vi "Main.vi"(8 "error in":errorcluster, 11 "Message Pump":refnum<class "Message Pump.lvclass">) -> (0 "error out":errorcluster, 3 "Message Pump out":refnum<class "Message Pump.lvclass">)   [LabVIEW 2023, in "Message Pump.lvclass"]
uses:
  Message Pump.lvclass
  C:/Program Files (x86)/National Instruments/LabVIEW 2023/vi.lib/addons/_Workers/Library/Classes/Worker/Worker.lvclass
  <vilib>/addons/_Workers/Library/Classes/Message Queue/Message Queue.lvclass
  <vilib>/addons/_Workers/Library/Case Label.ctl
  Message Pump.lvclass/Message Pump.ctl
  Initialization Data.ctl
  <vilib>/Utility/error.llb/Error Cluster From Error Code.vi
  <vilib>/addons/_Workers/Library/Classes/Message/Enqueue Message to Queue - Silent Mode.vi
  <vilib>/ErrorRing/Error Ring.xnode
  <vilib>/addons/_Workers/Library/Classes/Worker/Worker.lvclass
  <vilib>/addons/_Workers/Library/Workers.lvlib
  <vilib>/addons/_Workers/Library/Classes/Message/Message.lvclass
  C:/Program Files (x86)/National Instruments/LabVIEW 2023/vi.lib/addons/_Workers/Library/Classes/Workers Object/Workers Object.lvclass
  C:/Projects/DPP Workers/Workers/Message Pump/Message Pump.lvclass
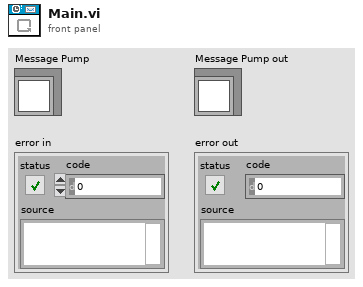
[diagram p1: front panel]
types:
  T1 = typedef "Message Pump.lvclass/Initialization Data.ctl" = cluster{"Caller Queue":refnum<class "Message Queue.lvclass">}
  T2 = typedef "WORKERS.lvlib/Case Label.ctl" = string
  T3 = typedef "Workers.lvlib/Case Label.ctl" = string
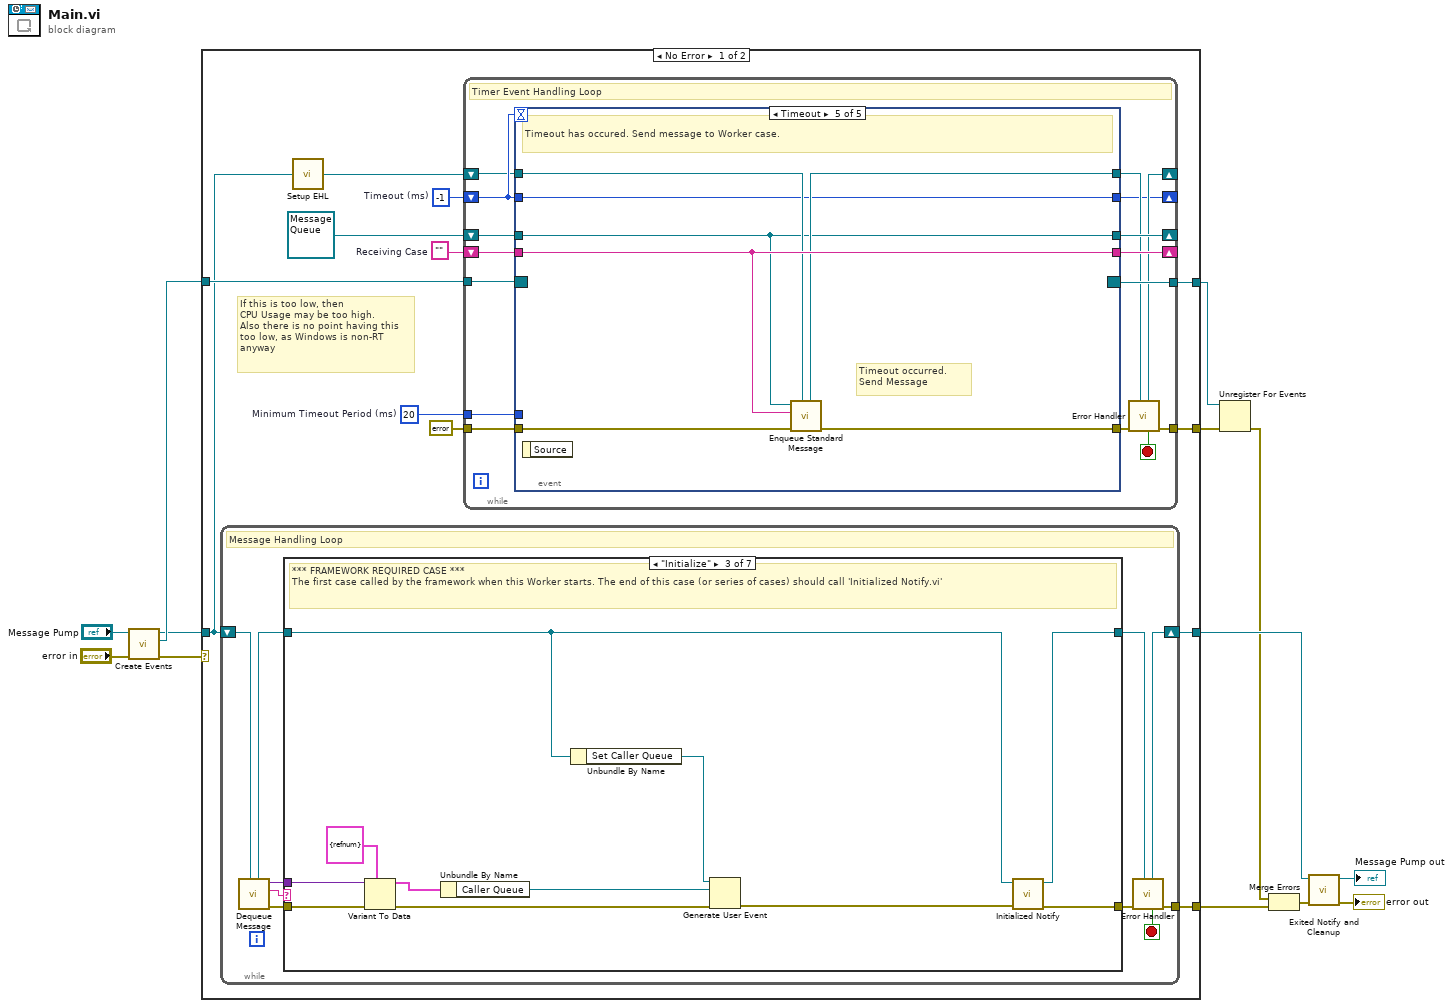
[diagram p0: block diagram]
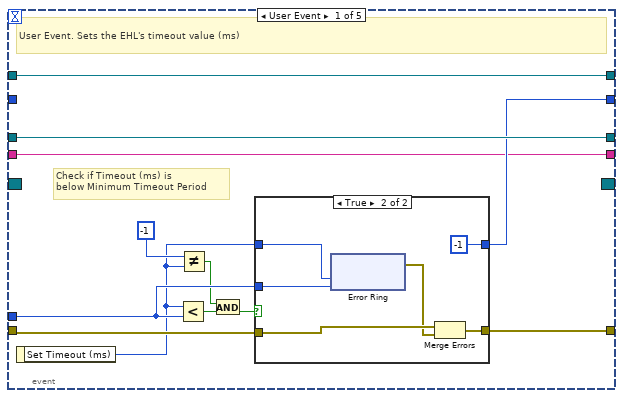
[diagram p2: hidden frame]
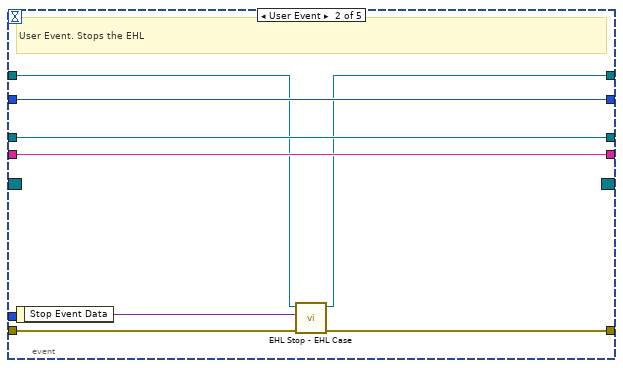
[diagram p4: hidden frame]
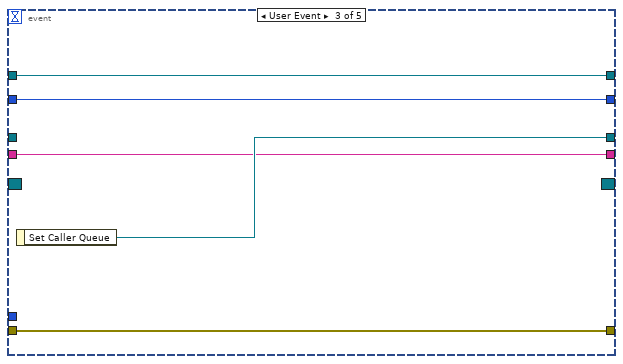
[diagram p5: hidden frame]
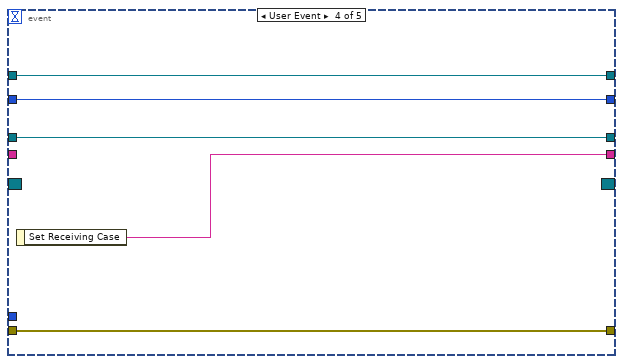
[diagram p6: hidden frame]
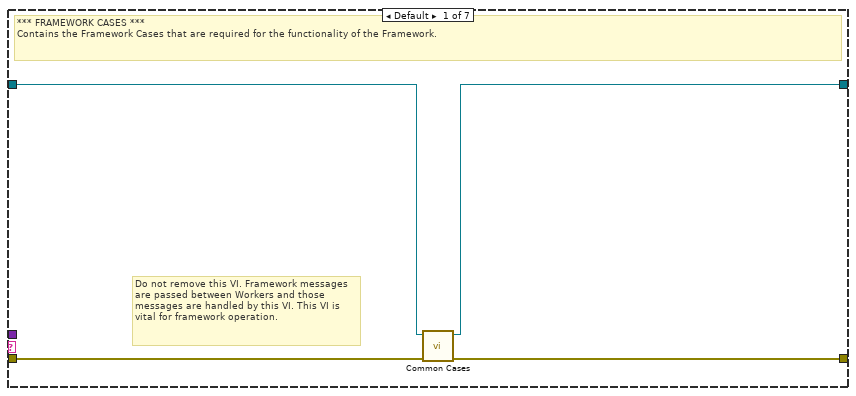
[diagram p7: hidden frame]
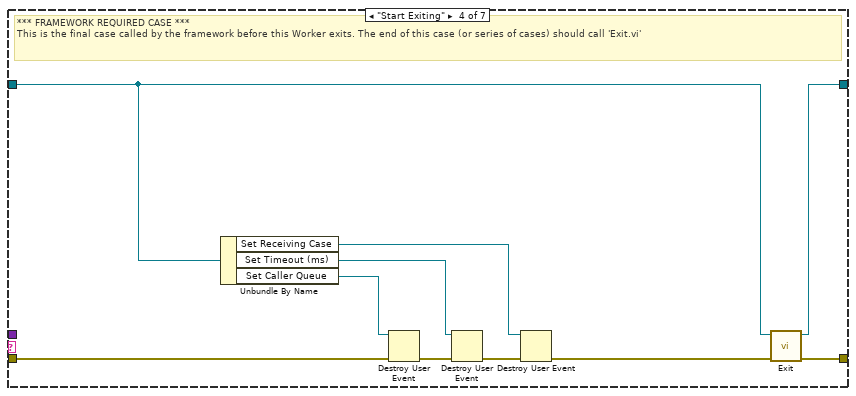
[diagram p9: hidden frame]
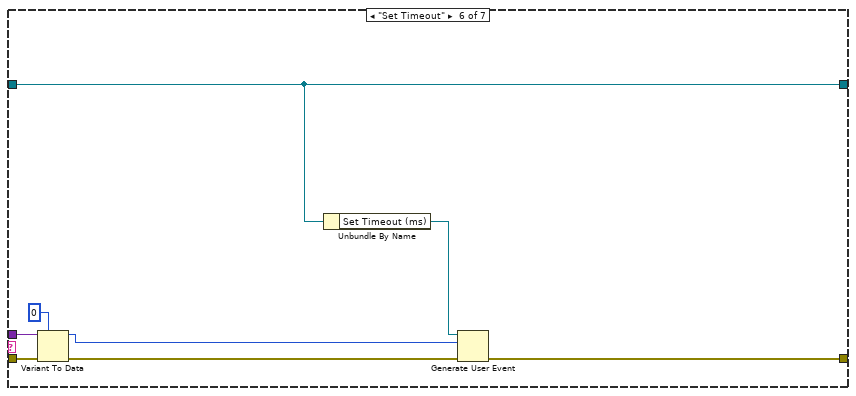
[diagram p11: hidden frame]
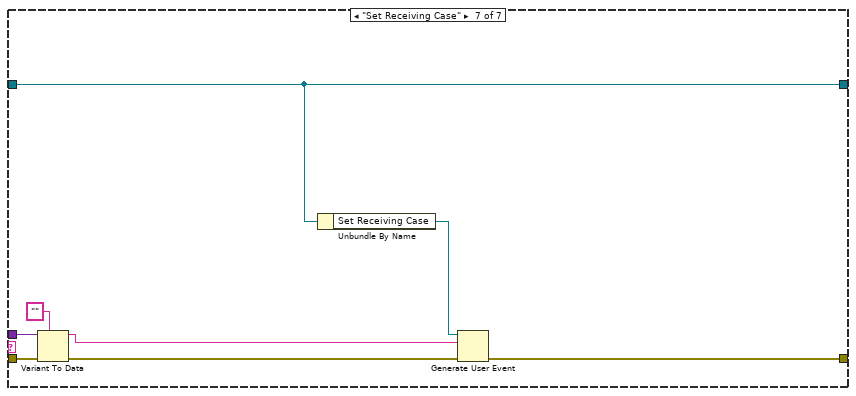
[diagram p12: hidden frame]
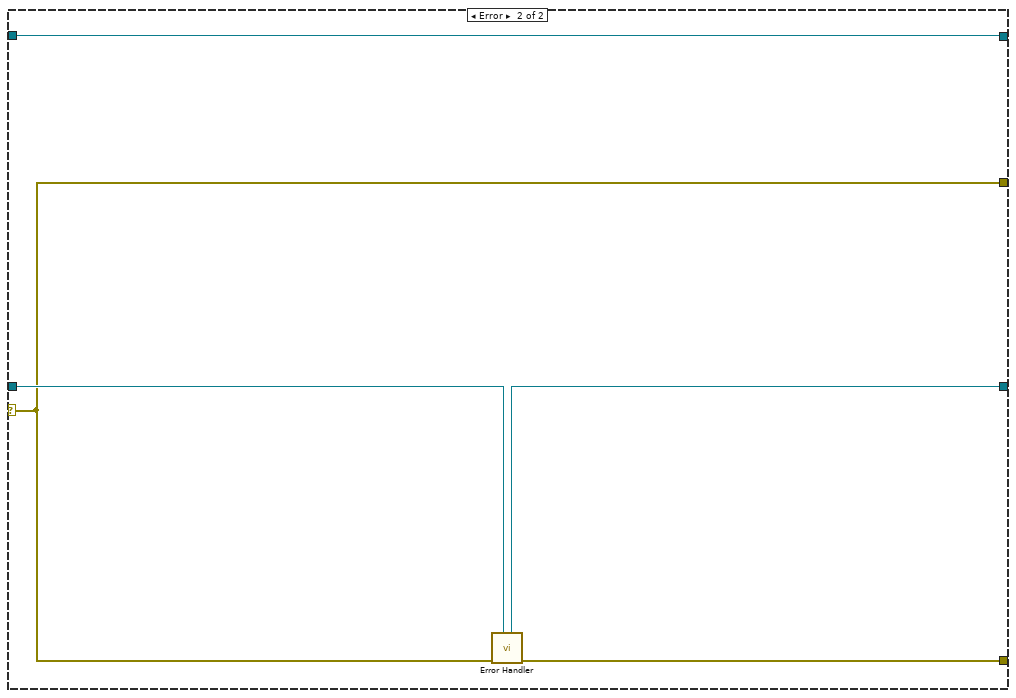
[diagram p13: hidden frame]
diagram:
  n1 = call "Create Events.vi"("error in"="error in", "Message Pump in"="Message Pump") -> ("error out"=w8:errorcluster, "Event Registration Refnum"=w9:refnum<event-registration>, "Message Pump out"=w4:refnum<class "Message Pump.lvclass">)  [unwired: 6 in]
  n2 = case shown="No Error" w8 {
    tunnel: w4 -> [w15 w153]
    tunnel: [w25 w154] -> w12
    tunnel: [w24 w152] -> w13
    selector: w8 -> [_ w151]
    tunnel: [w17 w151] -> w2
    tunnel: [w19 w150] -> w3
    tunnel: w9 -> [w18 w150]
    frame No Error {
      w23 = T2 ""  # Receiving Case
      w22 = 20  # Minimum Timeout Period (ms)
      w21 = -1  # Timeout (ms)
      # "If this is too low, then \nCPU Usage may be too high.\nAlso there is no point having this\ntoo low, as Windows is non-RT\nanyway"
      n3 = while {
        shift-right: [w102] -> w24
        shift-left: w15 -> [w104]
        tunnel: [w103] -> w25
        stop <- w95 stop-if-true
        # "Message Handling Loop"
        n4 = call-dynamic "Dequeue Message.vi"("Worker"=w104) -> ("error out"=w101:errorcluster, "Case out"=w96:string, "Data out"=w97:variant, "Worker out"=w99:refnum<class "Message Pump.lvclass">)  [unwired: 6 in, 1 out]
        n5 = case "WORKERS MHL Case Structure (DO NOT CHANGE LABEL NAME)" shown="\"Initialize\"" w96 {
          tunnel: w101 -> [w108 w109 w119 w124 w132 w141 w149]
          tunnel: [w107 w109 w121 w131 w132 w137 w146] -> w100
          tunnel: w99 -> [w106 w110 w113 w122 w133 w135 w144]
          tunnel: [w105 w110 w120 w130 w133 w135 w144] -> w98
          tunnel: w97 -> [_ _ w118 _ _ w140 w148]
          frame Default {
            # "Do not remove this VI. Framework messages are passed between Workers and those messages are handled by this VI. This VI is vital for framework operation."
            # "*** FRAMEWORK CASES ***\nContains the Framework Cases that are required for the functionality of the Framework."
            n6 = call-dynamic "Common Cases.vi"("error in"=w108, "Worker in"=w106) -> ("error out"=w107:errorcluster, "Worker out"=w105:refnum<class "Message Pump.lvclass">)  [unwired: 8 in]
          }
          frame "------ FRAMEWORK REQUIRED CASES ------" {
            # "Start of Framework Required Cases"
          }
          frame "Initialize" {
            # "*** FRAMEWORK REQUIRED CASE ***\nThe first case called by the framework when this Worker starts. The end of this case (or series of cases) should call 'Initialized Notify.vi'"
            n7 = Variant To Data(error in=w119, type=T1 {"Caller Queue"=refnum} ("Initialize Data"), Variant=w118) -> (data=w116:T1, error out=w115:errorcluster)
            n8 = Unbundle By Name(w116) -> ("Caller Queue"=w111:refnum<class "Message Queue.lvclass">)
            n9 = Unbundle By Name(w113) -> ("Set Caller Queue"=w114:refnum<user-event>)
            n10 = Generate User Event(user event=w114, event data cluster=w111, error in=w115) -> (error out=w112:errorcluster)  [unwired: 1 in, 1 out]
            n11 = call-dynamic "Initialized Notify.vi"("error in"=w112, "Worker"=w113) -> ("error out"=w121:errorcluster, "dup Worker out"=w120:refnum<class "Message Pump.lvclass">)  [unwired: 8 in]
          }
          frame "Start Exiting" {
            # "*** FRAMEWORK REQUIRED CASE ***\nThis is the final case called by the framework before this Worker exits. The end of this case (or series of cases) should call 'Exit.vi'"
            n12 = Unbundle By Name(w122) -> ("Set Receiving Case"=w129:refnum<user-event>, "Set Timeout (ms)"=w125:refnum<user-event>, "Set Caller Queue"=w126:refnum<user-event>)
            n13 = Destroy User Event(user event=w126, error in=w124) -> (error out=w127:errorcluster)
            n14 = Destroy User Event(user event=w125, error in=w127) -> (error out=w128:errorcluster)
            n15 = Destroy User Event(user event=w129, error in=w128) -> (error out=w123:errorcluster)
            n16 = call-dynamic "Exit.vi"("error_in"=w123, "Worker"=w122) -> ("error out"=w131:errorcluster, "dup Worker out"=w130:refnum<class "Message Pump.lvclass">)  [unwired: 8 in]
          }
          frame "-----------------------------------------------" {
            # "End of Framework Required Cases"
          }
          frame "Set Timeout" {
            n17 = Variant To Data(error in=w141, type=0 ("Timeout (ms)"), Variant=w140) -> (data=w134:i32, error out=w136:errorcluster)
            n18 = Unbundle By Name(w135) -> ("Set Timeout (ms)"=w138:refnum<user-event>)
            n19 = Generate User Event(user event=w138, event data cluster=w134, error in=w136) -> (error out=w137:errorcluster)  [unwired: 1 in, 1 out]
          }
          frame "Set Receiving Case" {
            n20 = Variant To Data(error in=w149, type=T2 "" ("Receiving Case"), Variant=w148) -> (data=w143:T2, error out=w145:errorcluster)
            n21 = Unbundle By Name(w144) -> ("Set Receiving Case"=w147:refnum<user-event>)
            n22 = Generate User Event(user event=w147, event data cluster=w143, error in=w145) -> (error out=w146:errorcluster)  [unwired: 1 in, 1 out]
          }
        }
        n23 = call-dynamic "Error Handler.vi"("Worker"=w98, "error_in"=w100) -> ("error out"=w103:errorcluster, "Stop Loop"=w95:bool, "Worker out"=w102:refnum<class "Message Pump.lvclass">)  [unwired: 7 in]
      }
      n24 = call-dynamic "Setup EHL.vi"("Worker"=w15) -> ("Worker out"=w14:refnum<class "Message Pump.lvclass">)  [unwired: 14 in]
      n25 = while "Event Handling Loop" {
        shift-right: [w26] -> _
        shift-left: w21 -> [w40]
        tunnel: errorcluster {"status"=FALSE, "code"=0, "source"=""} ("error IO") -> [w41]
        tunnel: [w31] -> w17
        shift-right: [w37] -> _
        shift-left: refnum<class "Message Queue.lvclass"> refnum ("Worker Queue") -> [w38]
        shift-right: [w36] -> _
        shift-left: w23 -> [w39]
        tunnel: w18 -> [w35]
        tunnel: [w34] -> w19
        tunnel: w22 -> [w33]
        shift-right: [w28] -> _
        shift-left: w14 -> [w30]
        stop <- w27 stop-if-true
        # "Timer Event Handling Loop"
        n26 = event shown="[4] Timeout" {
          selector: w35 -> [_ _ _ _ _]
          dyn-events: [_ _ _ _ _] -> w34
          timeout: w40 -> [_ _ _ _ _]
          tunnel: w41 -> [w50 w77 w82 w87 w94]
          tunnel: [w51 w73 w82 w87 w92] -> w32
          tunnel: w40 -> [_ w76 w81 w86 w89]
          tunnel: [w48 w76 w81 w86 w89] -> w26
          tunnel: w39 -> [w42 w74 w78 _ w93]
          tunnel: [w53 w75 w79 w83 w88] -> w37
          tunnel: w38 -> [w53 w75 _ w83 w88]
          tunnel: [w42 w74 w78 w84 w93] -> w36
          tunnel: w33 -> [w49 _ _ _ _]
          tunnel: w30 -> [w43 w72 w80 w85 w91]
          tunnel: [w43 w71 w80 w85 w90] -> w29
          event User Event {
            # "Check if Timeout (ms) is\nbelow Minimum Timeout Period"
            # "User Event. Sets the EHL's timeout value (ms)"
            n27 = event-data() -> ("Set Timeout (ms)"=w45:i32)  [unwired: 1 in]
            n28 = Less?(x=w45, y=w49) -> (x < y?=w52:bool)
            n29 = Not Equal?(x=-1 ("Set Timeout (ms)"), y=w45) -> (x != y?=w44:bool)
            n30 = And(x=w44, y=w52) -> (x .and. y?=w47:bool)
            n31 = case shown="True" w47 {
              tunnel: [w55 w59] -> w51
              tunnel: w50 -> [w55 w60]
              tunnel: w45 -> [w54 w57]
              tunnel: w49 -> [_ w56]
              tunnel: [w54 -1 ("Set Timeout (ms)")] -> w48
              frame False {
              }
              frame True {
                n32 = xnode "Error Ring"("parameter 0"=w57, "parameter 1"=w56) -> ("error out"=w58:errorcluster)
                n33 = Merge Errors(w60, w58) -> (w59:errorcluster)
              }
            }
          }
          event User Event {
            # "User Event. Stops the EHL"
            n34 = event-data() -> ("Stop Event Data"=w70:variant)  [unwired: 1 in]
            n35 = call <vilib>:"EHL Stop - EHL Case.vi"("error in"=w77, "Stop Event Data"=w70, "Worker"=w72) -> ("error out"=w73:errorcluster, "Worker out"=w71:refnum<class "Message Pump.lvclass">)  [unwired: 7 in]
          }
          event User Event {
            n36 = event-data() -> ("Set Caller Queue"=w79:refnum<class "Message Queue.lvclass">)  [unwired: 1 in]
          }
          event User Event {
            n37 = event-data() -> ("Set Receiving Case"=w84:T3)  [unwired: 1 in]
          }
          event Timeout {
            # "Timeout occurred.\nSend Message"
            # "Timeout has occured. Send message to Worker case."
            n38 = event-data() -> ()  [unwired: 1 in, 1 out]
            n39 = call-poly <vilib>:"Enqueue Standard Message.vi"("Worker"=w91, "error in"=w94, "Case Label"=w93, "Message Queue"=w88) -> ("error out"=w92:errorcluster, "dup Worker out"=w90:refnum<class "Message Pump.lvclass">)  [unwired: 5 in, 1 out]
          }
        }
        n40 = call-dynamic "Error Handler.vi"("Worker"=w29, "error_in"=w32) -> ("error out"=w31:errorcluster, "Stop Loop"=w27:bool, "Worker out"=w28:refnum<class "Message Pump.lvclass">)  [unwired: 7 in]
      }
    }
    frame Error {
      n41 = call-dynamic "Error Handler.vi"("Worker"=w153, "error_in"=w151) -> ("error out"=w154:errorcluster, "Worker out"=w152:refnum<class "Message Pump.lvclass">)  [unwired: 7 in, 1 out]
    }
  }
  n42 = Unregister For Events(event registration refnum=w3, error in=w2) -> (error out=w1:errorcluster)
  n43 = Merge Errors(w1, w12) -> (w11:errorcluster)
  n44 = call-dynamic "Exited Notify and Cleanup.vi"("error_in"=w11, "Worker"=w13) -> ("error out"=→"error out":errorcluster, "dup Worker out"=→"Message Pump out":refnum<class "Message Pump.lvclass">)  [unwired: 8 in]
